vi "Read msgQ.vi"(8 "error in":errorcluster, 11 "MsgQ enum":T1) -> (0 "error out":errorcluster, 2 "Message Received Parameters":variant, 3 "Message Received String":string, 5 "Message Recieved?":bool)   [LabVIEW 2013, in "Main MsgQ.lvlib"]
doc: "Reads the next message (string and varian parameter) from the specified message queue.\nReturns a true value if a message is found, doesnt wait for new messages."
uses:
  Main MsgQ.lvlib
  MsgQ Loops enum.ctl
  Common/Interloop MessageQ/Message que instance modes enum.ctl
  Common/Interloop MessageQ/Interloop MessageQ.lvlib
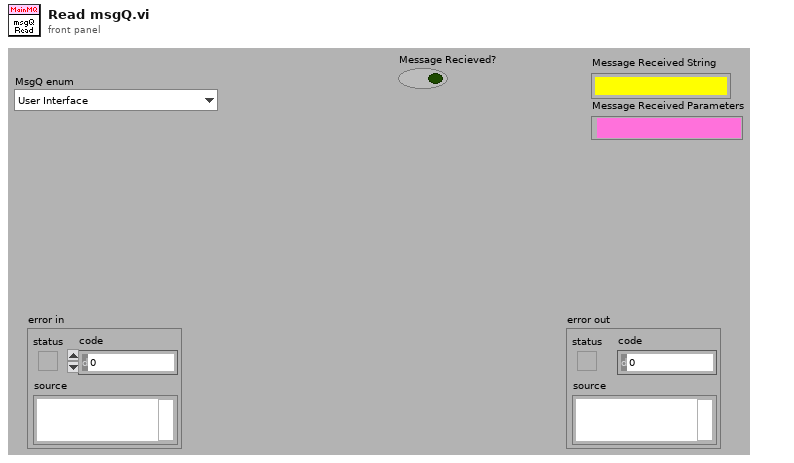
[diagram p1: front panel]
types:
  T1 = typedef "Main MsgQ.lvlib/MsgQ Loops enum.ctl" = enum16{"User Interface", "Image Acq"}
  T2 = typedef "Interloop MessageQ.lvlib/Message que instance modes enum.ctl" = enum16{"Initialize", "Broadcast Message", "Send Message", "Read Message", "Kill"}
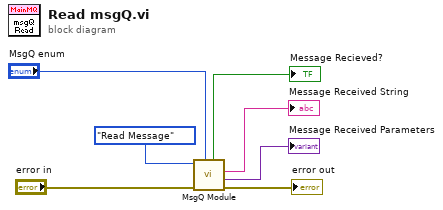
[diagram p0: block diagram]
diagram:
  n1 = call "MsgQ Module.vi"("MsgQ enum"="MsgQ enum", "error in (no error)"="error in", "Mode"=Message_que_instance_modes_enum."Read Message") -> ("error out"=→"error out":errorcluster, "Message Received Parameters"=→"Message Received Parameters":variant, "Message Received String"=→"Message Received String":string, "Message Recieved?"=→"Message Recieved?":bool)  [unwired: 5 in]
